vi "Edit Saquencer Array.vi"(11 "Sys Ini Path":path=path "D:/LABVIEW/SEQUENSER_SNA/Ver_12/INI/SysConfig.ini") -> ()   [LabVIEW 2018]
uses:
  Ctl/Step Type.ctl
  Ctl/MultiColumn Sequencer Table.ctl
  <vilib>/Utility/miscctls.llb/LVRowAndColumnUnsignedTypeDef.ctl
  <vilib>/Utility/miscctls.llb/LVRowAndColumnTypeDef.ctl
  Ctl/Test Step.ctl
  Ctl/Test Result.ctl
  Ctl/Sequencer Array.vi
  Ctl Main/Global Variable.vi
  <vilib>/Utility/config.llb/Read Key (String).vi
  <vilib>/Utility/config.llb/Read Key (U32).vi
  <vilib>/Utility/config.llb/Read Key (Double).vi
  <vilib>/Utility/config.llb/Read Key (Boolean).vi
  <vilib>/Utility/config.llb/Write Key (U32).vi
  <vilib>/Utility/config.llb/Write Key (String).vi
  <vilib>/Utility/config.llb/Write Key (Double).vi
  <vilib>/Utility/config.llb/Write Key (Boolean).vi
  <vilib>/Utility/config.llb/Write Key (I32).vi
  <vilib>/Utility/config.llb/NI_LVConfig.lvlib
panel:
  out "Sequencer File":string
  in  "Config":string="***"
  in  "Board":string="***"
  in  "Customer":string="***"
  in  "Sequencer\nExtend":bool
  in  "Save To File":bool
  in  "Load from File":bool
  in  "Value Nominal":dbl step=0.1 format="%#.3g"
  out "Row Selected":i16
  in  "Limits Calculate":bool
  in  "Test Sequencer":T1
  in  "New Step":bool
  in  "Measure Units":string
  in  "Remove Step":bool
  in  "Replace Step":bool
  in  "Insert Step":bool
  in  "Clear Array":bool
  in  "Exit Button":bool
  out "Steps":u16 max=500
  in  "Report":bool
  in  "Run/Skip":bool=TRUE
  in  "Parameters":string
  in  "Prc % (-)":i16=-5 min=-100 max=0 step=1
  in  "Prc % (+)":i16=5 min=0 max=100 step=1
  in  "Lower Limt":dbl step=0.1 format="%#.3g"
  in  "Upper Limt":dbl step=0.1 format="%#.3g"
  in  "Description":string
  in  "Step-ID":u16 max=255
  in  "Step Type":T2 items=["Label", "Settings", "Numeric", "String", "Boolean"]
  # "Step Editor"
  # "Nominal \nValue"
  # "Step Info"
  # "Measure Limits"
  # "File Operations"
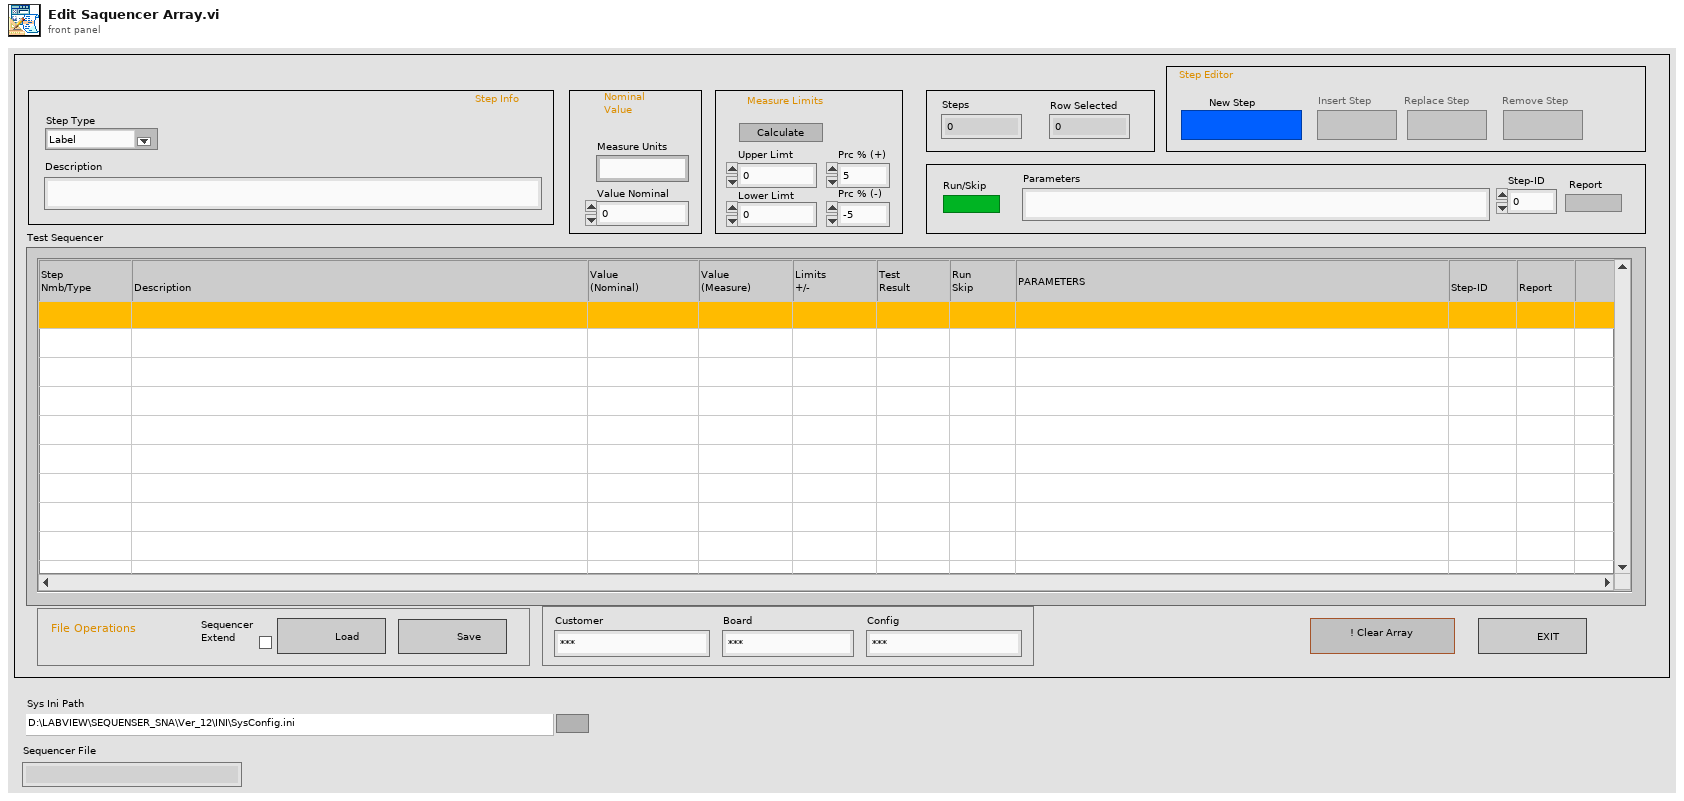
[diagram p1: front panel]
types:
  T1 = typedef "MultiColumn Sequencer Table.ctl" = i32
  T2 = typedef "Step Type.ctl" = u16
  T3 = typedef "LVRowAndColumnTypeDef.ctl" = cluster{"Row":i32, "Column":i32}
  T4 = typedef "LVRowAndColumnUnsignedTypeDef.ctl" = cluster{"Row":u32, "Column":u32}
  T5 = typedef "Test Step.ctl" = cluster{"Step ID":u16, "Step Description":string, "Step Type":u16, "Test Values":cluster{"Numeric Value":dbl, "Str Value":string, "Boolean Value":bool, "Upper Limit":dbl, "Lower Limit":dbl}, "Parameters":string, "Run/Skip":bool, "Test Result":T6, "Report":bool, "Measure Units":string}
  T6 = typedef "Test Result.ctl" = enum16{"Idle", "PASS", "FALSE"}
  T7 = enum8{"Enabled", "Disabled", "Disabled and Grayed Out"}
  T8 = enum16{"open", "replace", "create", "open or create", "replace or create", "replace or create with confirmation"}
  T9 = typedef "NI_LVConfig.lvlib/Config Data RefNum.ctl" = refnum<k1>
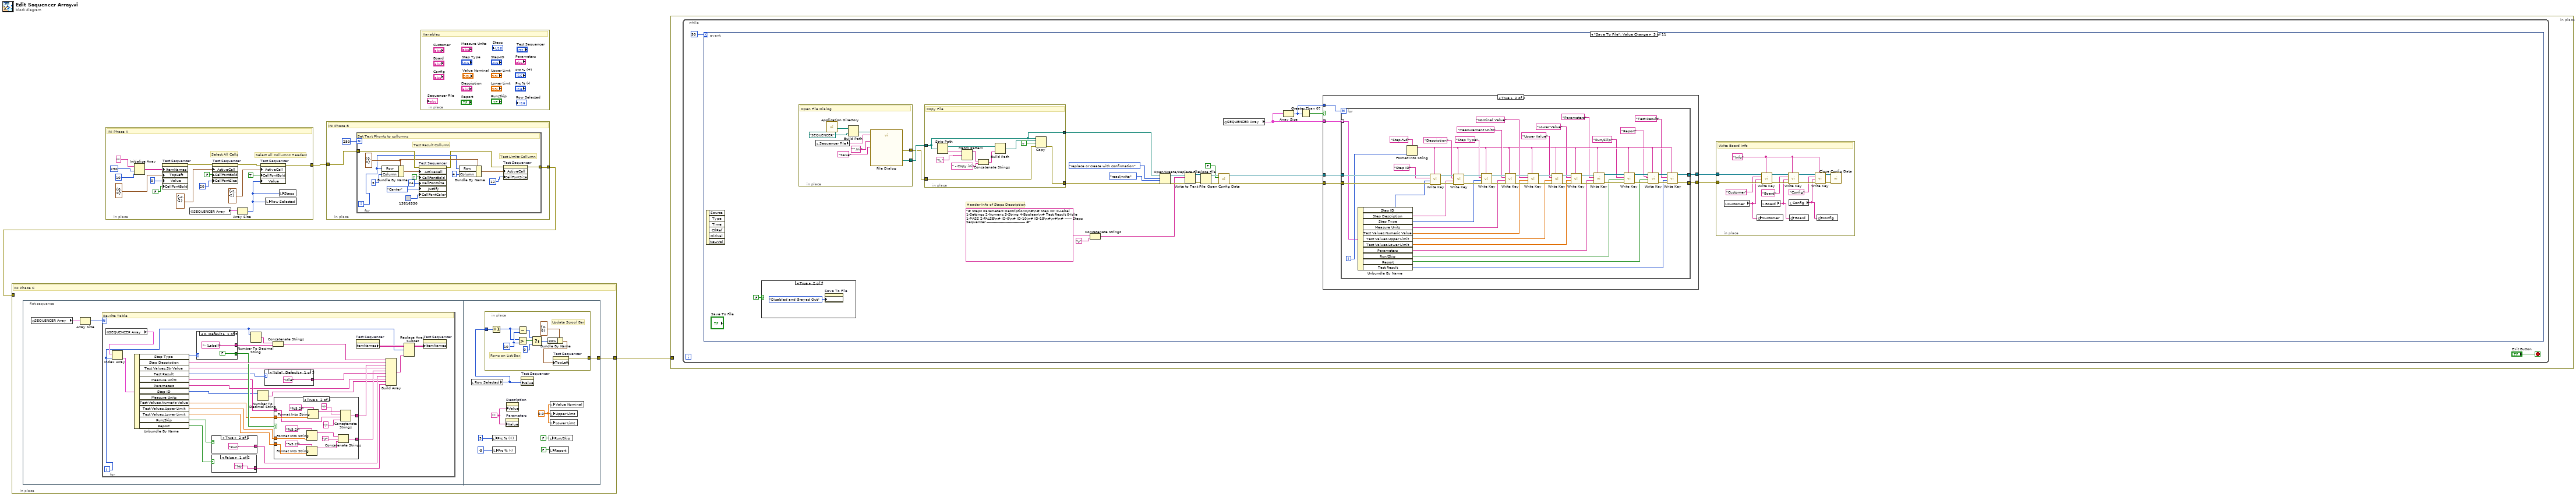
[diagram p0: block diagram]
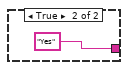
[diagram p2: hidden frame]
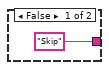
[diagram p3: hidden frame]
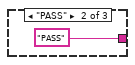
[diagram p4: hidden frame]
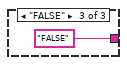
[diagram p5: hidden frame]
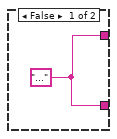
[diagram p6: hidden frame]
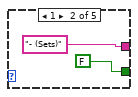
[diagram p7: hidden frame]
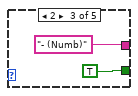
[diagram p8: hidden frame]
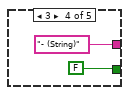
[diagram p9: hidden frame]
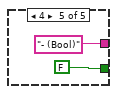
[diagram p10: hidden frame]
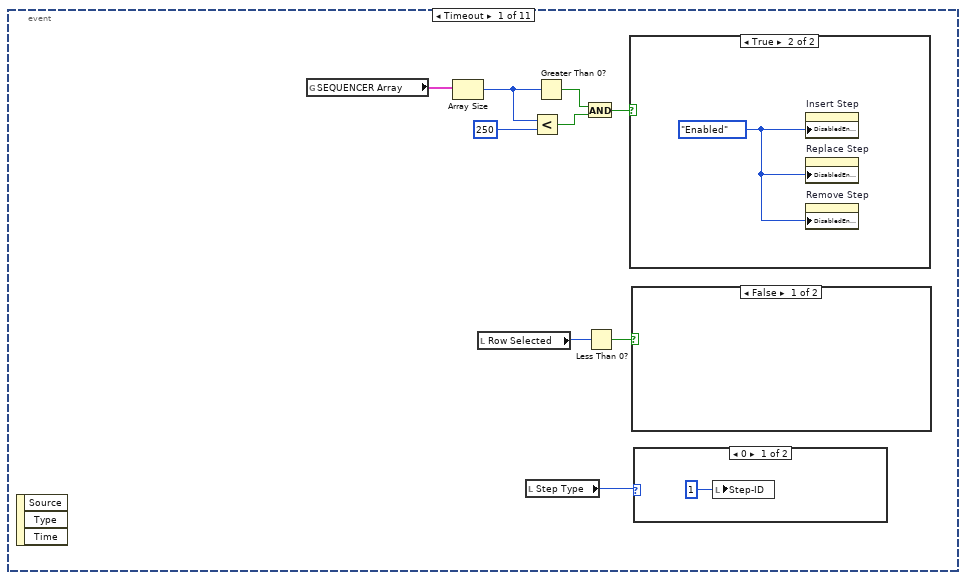
[diagram p11: hidden frame]
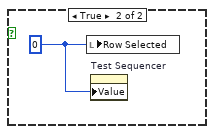
[diagram p13: hidden frame]
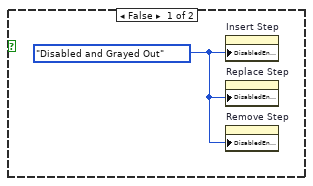
[diagram p14: hidden frame]
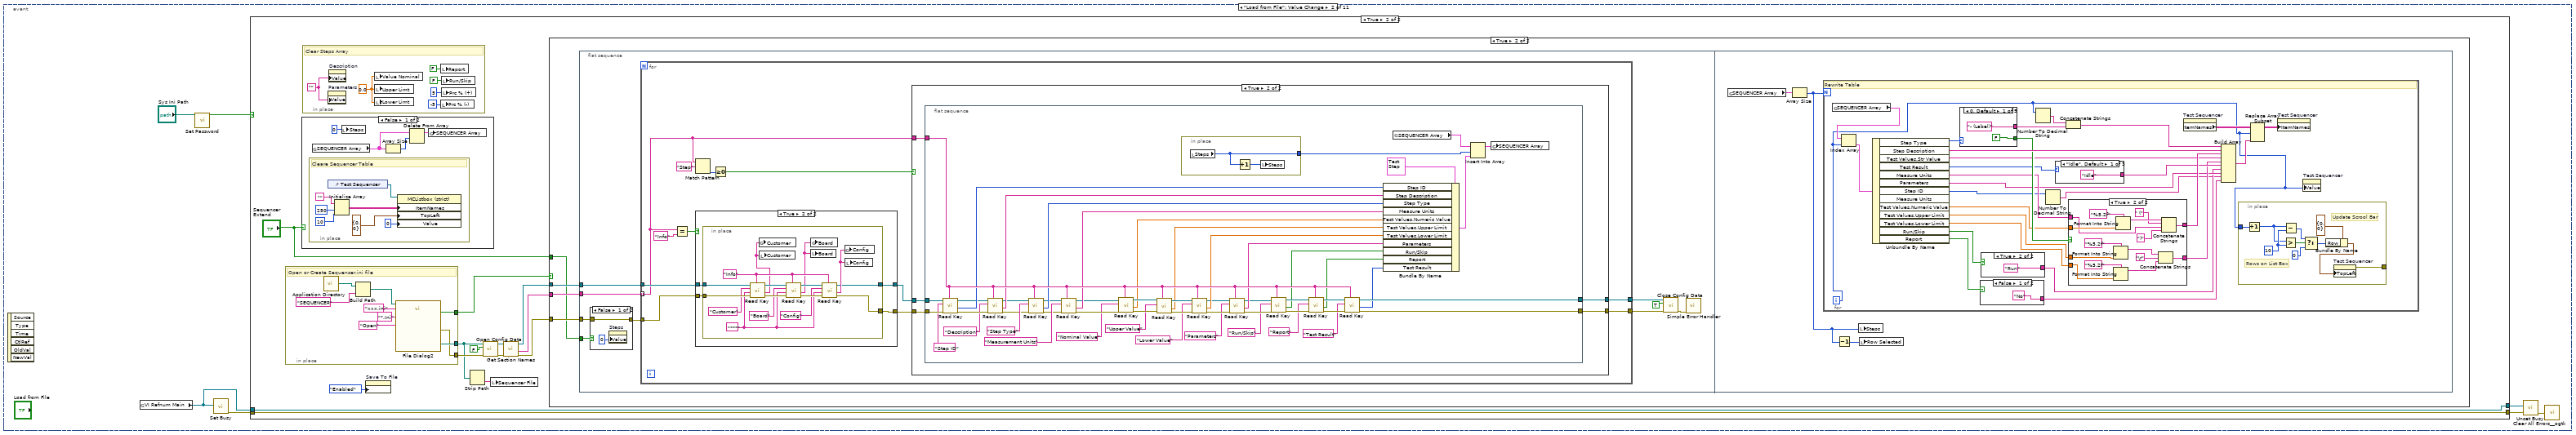
[diagram p15: hidden frame]
diagram:
  n1 = in-place {
    in-place-border: [w6] -> w3
    # "Select All Collumns Headers"
    # "Select All Cells"
    # "INI Phase A"
    n2 = Initialize Array("", 250 ("dimension size"), 10 ("dimension size")) -> (w18:string[][])
    n3 = property on="Test Sequencer" class="MCListbox (strict)"("ItemNames"=w18, "TopLeft"=T4 {"Row"=0, "Column"=0} ("Top Left Visible Cell"), "Value"=T1 0 ("Test Sequencer"), "CellFontBold"=FALSE ("Active Cell:Cell Font:Bold")) -> (error out=w13:errorcluster)  [unwired: 2 in, 1 out]
    n4 = global read "Sequencer Array.vi" "SEQUENCER Array"() -> (w5:T5[])
    n5 = property on="Test Sequencer" class="MCListbox (strict)"(error in=w13, "ActiveCell"=T3 {"Row"=-2, "Column"=-2} ("Active Cell:Active Cell"), "CellFontBold"=FALSE ("Active Cell:Cell Font:Bold"), "CellFontSize"=20 ("dimension size")) -> (error out=w7:errorcluster)  [unwired: 1 in, 1 out]
    n6 = Array Size(array=w5) -> (size(s)=w4:i32)
    n7 = property on="Test Sequencer" class="MCListbox (strict)"(error in=w7, "ActiveCell"=T3 {"Row"=-1, "Column"=-2} ("Active Cell:Active Cell"), "CellFontBold"=TRUE ("Active Cell:Cell Font:Bold"), "Value"=w4) -> (error out=w6:errorcluster)  [unwired: 1 in, 1 out]
    n8 = local write "Row Selected"(w4) -> ()
    n9 = local write "Steps"(w4) -> ()
  }
  n10 = in-place {
    in-place-border: w3 -> [w22]
    in-place-border: [w21] -> w2
    # "INI Phase B"
    n11 = for {
      N: 250 -> [_]
      tunnel: w22 -> [w35]
      tunnel: [w27] -> w21
      i -> [w28]
      w30 = T3 {"Row"=0, "Column"=0} ("Active Cell:Active Cell")
      # "Test Limits Collumn"
      # "Test Result Collumn"
      # "Set Text Phonts to collumns"
      n12 = Bundle By Name(cluster=w30, "Row"=w28, "Column"=5) -> (w37:T3)
      n13 = property on="Test Sequencer" class="MCListbox (strict)"(error in=w35, "ActiveCell"=w37, "CellFontBold"=TRUE ("Active Cell:Cell Font:Bold"), "CellFontSize"=u32 24 ("Active Cell:Cell Font:Size"), "Justify"=enum16{"Left", "Center", "Right"}."Center" ("Active Cell:Cell Justification"), "CellFontColor"=u32 13816530) -> (error out=w26:errorcluster)  [unwired: 1 in, 1 out]
      n14 = Bundle By Name(cluster=w30, "Row"=w28, "Column"=4) -> (w29:T3)
      n15 = property on="Test Sequencer" class="MCListbox (strict)"(error in=w26, "ActiveCell"=w29, "CellFontSize"=12 ("Column")) -> (error out=w27:errorcluster)  [unwired: 1 in, 1 out]
    }
  }
  n16 = in-place {
    in-place-border: w2 -> [_]
    in-place-border: [w38] -> w1
    # "INI Phase C"
    n17 = flat-sequence {
      tunnel: [w108] -> w38
      frame #0 {
        n18 = global read "Sequencer Array.vi" "SEQUENCER Array"() -> (w40:T5[])
        n19 = Array Size(array=w40) -> (size(s)=w39:i32)
        n20 = for {
          N: w39 -> [_]
          i -> [w63]
          # "Revrite Table"
          n21 = global read "Sequencer Array.vi" "SEQUENCER Array"() -> (w68:T5[])
          n22 = Index Array(array=w68, index=w63) -> (element=w49:T5)
          n23 = Unbundle By Name(w49) -> ("Step Type"=w67:u16, "Step Description"=w59:string, "Test Values.Str Value"=w55:string, "Test Result"=w54:T6, "Measure Units"=w52:string, "Parameters"=w48:string, "Step ID"=w50:u16, "Test Values.Numeric Value"=w57:dbl, "Test Values.Upper Limit"=w47:dbl, "Test Values.Lower Limit"=w46:dbl, "Run/Skip"=w45:bool, "Report"=w44:bool)  [unwired: 1 out]
          n24 = case shown="0, Default" w67 {
            tunnel: ["- (Label)" "- (Sets)" "- (Numb)" "- (String)" "- (Bool)"] -> w61
            tunnel: [FALSE FALSE TRUE FALSE FALSE] -> w58
            frame 0, Default {
            }
            frame 1 {
            }
            frame 2 {
            }
            frame 3 {
            }
            frame 4 {
            }
          }
          n25 = case shown="False" w44 {
            tunnel: ["No" "Yes"] -> w42
            frame False {
            }
            frame True {
            }
          }
          n26 = case shown="True" w45 {
            tunnel: ["Skip" "Run"] -> w43
            frame False {
            }
            frame True {
            }
          }
          n27 = Number To Decimal String(number=w63) -> (decimal integer string=w62:string)  [unwired: 1 in]
          n28 = Number To Decimal String(number=w50) -> (decimal integer string=w41:string)  [unwired: 1 in]
          n29 = case shown="\"Idle\", Default" w54 {
            tunnel: ["Idle" "PASS" "FALSE"] -> w53
            frame "Idle", Default {
            }
            frame "PASS" {
            }
            frame "FALSE" {
            }
          }
          n30 = Concatenate Strings(w62, w61) -> (w60:string)
          n31 = case shown="True" w58 {
            tunnel: [w76 w85] -> w51
            tunnel: [w76 w82] -> w56
            tunnel: w57 -> [_ w80]
            tunnel: w47 -> [_ w79]
            tunnel: w46 -> [_ w78]
            tunnel: w52 -> [_ w77]
            frame False {
              w76 = "..."
            }
            frame True {
              n32 = Format Into String(format string="%5.2f", w79) -> (resulting string=w87:string)  [unwired: 2 in, 1 out]
              n33 = Format Into String(format string="%5.2f", w78) -> (resulting string=w86:string)  [unwired: 2 in, 1 out]
              n34 = Format Into String(format string="%5.2f", w80) -> (resulting string=w84:string)  [unwired: 2 in, 1 out]
              n35 = Concatenate Strings(w87, "\r", w86) -> (w85:string)
              n36 = Concatenate Strings(w84, "(", w77, ")") -> (w82:string)
            }
          }
          n37 = property on="Test Sequencer" class="MCListbox (strict)"() -> ("ItemNames"=w66:string[][])  [unwired: 2 in, 2 out]
          n38 = Build Array(w60, w59, w56, w55, w51, w53, w43, w48, w41, w42) -> (w64:string[])
          n39 = Replace Array Subset(array=w66, new element=w64, index (row)=w63) -> (w65:string[][])  [unwired: 1 in]
          n40 = property on="Test Sequencer" class="MCListbox (strict)"("ItemNames"=w65) -> ()  [unwired: 2 in, 2 out]
        }
      }
      frame #1 {
        w106 = 0.0
        w107 = ""
        n41 = local read "Row Selected"() -> (w109:i16)
        n42 = in-place {
          in-place-border: w109 -> [w113]
          in-place-border: [w110] -> w108
          w115 = 10 ("y")
          # "Update Scrool Bar"
          # "Rows on List Box"
          n43 = Increment(x=w113) -> (x+1=w112:i16)
          n44 = Greater?(x=w112, y=w115) -> (0:w118:bool)
          n45 = Subtract(x=w112, y=w115) -> (x-y=w116:i32)
          n46 = Select(t=w116, s=w118, f=0) -> (s? t:f=w114:i32)
          n47 = Bundle By Name(cluster=T4 {"Row"=0, "Column"=0} ("Top Left Visible Cell"), "Row"=w114) -> (w111:T4)
          n48 = property on="Test Sequencer" class="MCListbox (strict)"("TopLeft"=w111) -> (error out=w110:errorcluster)  [unwired: 2 in, 1 out]
        }
        n49 = local write "Prc % (+)"(5) -> ()
        n50 = local write "Prc % (-)"(i16 -5 ("Prc % (-)")) -> ()
        n51 = property on="Parameters" class="Str"("Value"=w107) -> ()  [unwired: 2 in, 2 out]
        n52 = property on="Description" class="Str"("Value"=w107) -> ()  [unwired: 2 in, 2 out]
        n53 = property on="Test Sequencer" class="MCListbox (strict)"("Value"=w109) -> ()  [unwired: 2 in, 2 out]
        n54 = local write "Run/Skip"(FALSE ("Run/Skip")) -> ()
        n55 = local write "Report"(FALSE ("Report")) -> ()
        n56 = local write "Value Nominal"(w106) -> ()
        n57 = local write "Upper Limt"(w106) -> ()
        n58 = local write "Lower Limt"(w106) -> ()
      }
    }
  }
  n59 = in-place {
    # "Variables"
  }
  n60 = in-place {
    in-place-border: w1 -> [_]
    n61 = while {
      stop <- "Exit Button" stop-if-true
      n62 = event shown="[2] \"Save To File\": Value Change" {
        selector: _ -> [_ _ _ _ _ _ _ _ _ _ _]
        dyn-events: _ -> [_ _ _ _ _ _ _ _ _ _ _]
        timeout: 50 -> [_ _ _ _ _ _ _ _ _ _ _]
        event Timeout {
          n63 = event-data() -> ()  [unwired: 1 in, 3 out]
          n64 = global read "Sequencer Array.vi" "SEQUENCER Array"() -> (w130:T5[])
          n65 = Array Size(array=w130) -> (size(s)=w129:i32)
          n66 = local read "Row Selected"() -> (w124:i16)
          n67 = local read "Step Type"() -> (w122:T2)
          n68 = Less?(x=w129, y=250) -> (x < y?=w126:bool)
          n69 = Greater Than 0?(x=w129) -> (x > 0?=w127:bool)
          n70 = And(x=w127, y=w126) -> (x .and. y?=w125:bool)
          n71 = Less Than 0?(x=w124) -> (x < 0?=w123:bool)
          n72 = case shown="True" w125 {
            frame False {
              w133 = T7."Disabled and Grayed Out" ("Disabled")
              n73 = property on="Insert Step" class="Bool"("DisabledEnum"=w133) -> ()  [unwired: 2 in, 2 out]
              n74 = property on="Replace Step" class="Bool"("DisabledEnum"=w133) -> ()  [unwired: 2 in, 2 out]
              n75 = property on="Remove Step" class="Bool"("DisabledEnum"=w133) -> ()  [unwired: 2 in, 2 out]
            }
            frame True {
              w134 = T7."Enabled" ("Disabled")
              n76 = property on="Insert Step" class="Bool"("DisabledEnum"=w134) -> ()  [unwired: 2 in, 2 out]
              n77 = property on="Replace Step" class="Bool"("DisabledEnum"=w134) -> ()  [unwired: 2 in, 2 out]
              n78 = property on="Remove Step" class="Bool"("DisabledEnum"=w134) -> ()  [unwired: 2 in, 2 out]
            }
          }
          n79 = case shown="False" w123 {
            frame False {
            }
            frame True {
              w132 = u16 0 ("Row Selected")
              n80 = local write "Row Selected"(w132) -> ()
              n81 = property on="Test Sequencer" class="MCListbox (strict)"("Value"=w132) -> ()  [unwired: 2 in, 2 out]
            }
          }
          n82 = case shown="0" w122 {
            frame 0 {
              n83 = local write "Step-ID"(1) -> ()
            }
            frame 1, Default {
            }
          }
        }
        event "Load from File": Value Change {
          n84 = event-data() -> ()  [unwired: 1 in, 6 out]
          n85 = global read "Global Variable.vi" "VI Refnum Main"() -> (w135:refnum<vi>)
          n86 = call "Set Password.vi"("Ini File"="Sys Ini Path") -> ("Password Ok"=w140:bool)  [unwired: 9 in, 1 out]
          n87 = call <vilib>:"Set Busy.vi"("VI reference (current VI)"=w135) -> ("error out"=w139:errorcluster)  [unwired: 9 in, 1 out]
          n88 = case shown="True" w140 {
            tunnel: w139 -> [w143 w145]
            tunnel: [w143 w145] -> w138
            tunnel: w135 -> [w142 w144]
            tunnel: [w142 w144] -> w136
            frame False {
            }
            frame True {
              n89 = in-place {
                in-place-border: [w366] -> w150
                in-place-border: [w365] -> w147
                in-place-border: [w364] -> w157
                # "Open or Create Sequenser.ini file"
                n90 = call <vilib>:"Application Directory.vi"() -> ("Application Directory"=w361:path)
                n91 = Build Path(base path=w361, name or relative path="SEQUENCER") -> (appended path=w363:path)
                n92 = call "File Dialog2"("start path"=w363, "button label"="Open", "default name"="xxx.ini", "pattern (all files)"="*.Ini") -> ("selected path"=w365:path, "exists"=w366:bool, "error out"=w364:errorcluster)  [unwired: 8 in, 1 out]
              }
              n93 = case shown="False" "Sequencer\nExtend" {
                frame False {
                  n94 = in-place "In Place Element Structure" {
                    # "Cleare Sequencer Table"
                    n95 = control-ref of="Test Sequencer"() -> (w163:refnum<vi>)
                    n96 = Initialize Array("", 250 ("dimension size"), 10 ("dimension size")) -> (w166:string[][])
                    n97 = property on="Property Node" class="MCListbox (strict)"(reference=w163, "ItemNames"=w166, "TopLeft"=T4 {"Row"=0, "Column"=0} ("Top Left Visible Cell"), "Value"=T1 0 ("Test Sequencer")) -> ()  [unwired: 1 in, 2 out]
                  }
                  n98 = global read "Sequencer Array.vi" "SEQUENCER Array"() -> (w159:T5[])
                  n99 = local write "Steps"(u16 0 ("Steps")) -> ()
                  n100 = Array Size(array=w159) -> (size(s)=w160:i32)
                  n101 = Delete From Array(array=w159, length=w160) -> (array with subset deleted=w161:T5[])  [unwired: 1 in, 1 out]
                  n102 = global write "Sequencer Array.vi" "SEQUENCER Array"(w161) -> ()
                }
                frame True {
                }
              }
              n103 = in-place {
                w355 = 0.0
                w354 = ""
                # "Clear Steps Array"
                n104 = property on="Parameters" class="Str"("Value"=w354) -> ()  [unwired: 2 in, 2 out]
                n105 = property on="Description" class="Str"("Value"=w354) -> ()  [unwired: 2 in, 2 out]
                n106 = local write "Value Nominal"(w355) -> ()
                n107 = local write "Upper Limt"(w355) -> ()
                n108 = local write "Lower Limt"(w355) -> ()
                n109 = local write "Report"(FALSE ("Report")) -> ()
                n110 = local write "Prc % (-)"(i16 -5 ("Prc % (-)")) -> ()
                n111 = local write "Run/Skip"(FALSE ("Run/Skip")) -> ()
                n112 = local write "Prc % (+)"(5) -> ()
              }
              n113 = property on="Save To File" class="Bool"("DisabledEnum"=T7."Enabled" ("Disabled")) -> ()  [unwired: 2 in, 2 out]
              n114 = Strip Path(path=w147) -> (name=w146:string)  [unwired: 1 out]
              n115 = call <vilib>:"Open Config Data.vi"("error in (no error)"=w157, "create file if necessary (T)"=FALSE, "configuration file path"=w147) -> ("error out"=w154:errorcluster, "refnum"=w155:T9)  [unwired: 6 in, 1 out]
              n116 = local write "Sequencer File"(w146) -> ()
              n117 = call <vilib>:"Get Section Names.vi"("error in (no error)"=w154, "refnum"=w155) -> ("error out"=w151:errorcluster, "section names"=w152:string[], "refnum out"=w153:T9)  [unwired: 7 in]
              n118 = case shown="True" w150 {
                tunnel: w153 -> [_ w172]
                tunnel: w152 -> [_ w171]
                tunnel: w151 -> [_ w170]
                tunnel: "Sequencer\nExtend" -> [_ w169]
                frame False {
                }
                frame True {
                  n119 = flat-sequence {
                    tunnel: w172 -> [w176]
                    tunnel: w171 -> [w181]
                    tunnel: w170 -> [w174]
                    tunnel: w169 -> [w173]
                    frame #0 {
                      n120 = case shown="False" w173 {
                        tunnel: [w183 w184] -> w175
                        tunnel: w174 -> [w183 w184]
                        frame False {
                          n121 = property on="Steps" class="DigNum (strict)"("Value"=u16 0 ("Steps")) -> ()  [unwired: 2 in, 2 out]
                        }
                        frame True {
                        }
                      }
                      n122 = for {
                        tunnel: w181 -> [w188] mode=indexing
                        tunnel: w175 -> [w193]
                        tunnel: [w196] -> w178
                        tunnel: [w195] -> w177
                        tunnel: w176 -> [w194]
                        n123 = Equal?(x=w188, y="Info") -> (x = y?=w189:bool)
                        n124 = Match Pattern(string=w188, regular expression="Step") -> (offset past match=w186:i32)  [unwired: 1 in, 3 out]
                        n125 = case shown="True" w189 {
                          tunnel: w194 -> [w259 w263]
                          tunnel: w193 -> [w258 w262]
                          tunnel: [w259 w261] -> w192
                          tunnel: [w258 w260] -> w191
                          frame False {
                          }
                          frame True {
                            n126 = in-place {
                              in-place-border: w263 -> [w275]
                              in-place-border: w262 -> [w274]
                              in-place-border: [w265] -> w261
                              in-place-border: [w264] -> w260
                              w269 = "***"
                              w273 = "Info"
                              n127 = call-poly <vilib>:"Read Key.vi"("section"=w273, "error in (no error)"=w274, "default value"=w269, "key"="Customer", "refnum"=w275) -> ("error out"=w278:errorcluster, "value"=w266:string, "refnum out"=w276:T9)  [unwired: 3 in, 1 out]
                              n128 = global write "Global Variable.vi" "Customer"(w266) -> ()
                              n129 = local write "Customer"(w266) -> ()
                              n130 = call-poly <vilib>:"Read Key.vi"("section"=w273, "error in (no error)"=w278, "default value"=w269, "key"="Board", "refnum"=w276) -> ("error out"=w279:errorcluster, "value"=w268:string, "refnum out"=w277:T9)  [unwired: 3 in, 1 out]
                              n131 = global write "Global Variable.vi" "Board"(w268) -> ()
                              n132 = local write "Board"(w268) -> ()
                              n133 = call-poly <vilib>:"Read Key.vi"("section"=w273, "error in (no error)"=w279, "default value"=w269, "key"="Config", "refnum"=w277) -> ("error out"=w264:errorcluster, "value"=w267:string, "refnum out"=w265:T9)  [unwired: 3 in, 1 out]
                              n134 = global write "Global Variable.vi" "Config"(w267) -> ()
                              n135 = local write "Config"(w267) -> ()
                            }
                          }
                        }
                        n136 = Greater Or Equal To 0?(x=w186) -> (x >= 0?=w185:bool)
                        n137 = case shown="True" w185 {
                          tunnel: [w198 w203] -> w196
                          tunnel: [w197 w202] -> w195
                          tunnel: w192 -> [w198 w201]
                          tunnel: w191 -> [w197 w200]
                          tunnel: w188 -> [_ w199]
                          frame False {
                          }
                          frame True {
                            n138 = flat-sequence {
                              tunnel: [w254] -> w202
                              tunnel: [w255] -> w203
                              tunnel: w199 -> [w251]
                              tunnel: w200 -> [w252]
                              tunnel: w201 -> [w253]
                              frame #0 {
                                n139 = call-poly <vilib>:"Read Key.vi"("section"=w251, "error in (no error)"=w252, "key"="Step ID", "refnum"=w253) -> ("error out"=w243:errorcluster, "value"=w245:u32, "refnum out"=w244:T9)  [unwired: 4 in, 1 out]
                                n140 = call-poly <vilib>:"Read Key.vi"("section"=w251, "error in (no error)"=w243, "key"="Description", "refnum"=w244) -> ("error out"=w238:errorcluster, "value"=w241:string, "refnum out"=w239:T9)  [unwired: 4 in, 1 out]
                                n141 = call-poly <vilib>:"Read Key.vi"("section"=w251, "error in (no error)"=w238, "key"="Step Type", "refnum"=w239) -> ("error out"=w234:errorcluster, "value"=w237:u32, "refnum out"=w235:T9)  [unwired: 4 in, 1 out]
                                n142 = call-poly <vilib>:"Read Key.vi"("section"=w251, "error in (no error)"=w234, "key"="Measurement Units", "refnum"=w235) -> ("error out"=w229:errorcluster, "value"=w233:string, "refnum out"=w232:T9)  [unwired: 4 in, 1 out]
                                n143 = call-poly <vilib>:"Read Key.vi"("section"=w251, "error in (no error)"=w229, "key"="Nominal Value", "refnum"=w232) -> ("error out"=w228:errorcluster, "value"=w223:dbl, "refnum out"=w231:T9)  [unwired: 4 in, 1 out]
                                n144 = call-poly <vilib>:"Read Key.vi"("section"=w251, "error in (no error)"=w228, "key"="Upper Value", "refnum"=w231) -> ("error out"=w227:errorcluster, "value"=w222:dbl, "refnum out"=w230:T9)  [unwired: 4 in, 1 out]
                                n145 = in-place {
                                in-place-border: [w257] -> w204
                                n146 = local read "Steps"() -> (w257:u16)
                                n147 = Increment(x=w257) -> (x+1=w256:u16)
                                n148 = local write "Steps"(w256) -> ()
                                }
                                n149 = call-poly <vilib>:"Read Key.vi"("section"=w251, "error in (no error)"=w227, "key"="Lower Value", "refnum"=w230) -> ("error out"=w219:errorcluster, "value"=w221:dbl, "refnum out"=w220:T9)  [unwired: 4 in, 1 out]
                                n150 = call-poly <vilib>:"Read Key.vi"("section"=w251, "error in (no error)"=w219, "key"="Parameters", "refnum"=w220) -> ("error out"=w213:errorcluster, "value"=w217:string, "refnum out"=w216:T9)  [unwired: 4 in, 1 out]
                                n151 = call-poly <vilib>:"Read Key.vi"("section"=w251, "error in (no error)"=w213, "key"="Run/Skip", "refnum"=w216) -> ("error out"=w212:errorcluster, "value"=w209:bool, "refnum out"=w215:T9)  [unwired: 4 in, 1 out]
                                n152 = call-poly <vilib>:"Read Key.vi"("section"=w251, "error in (no error)"=w212, "key"="Report", "refnum"=w215) -> ("error out"=w211:errorcluster, "value"=w206:bool, "refnum out"=w214:T9)  [unwired: 4 in, 1 out]
                                n153 = call-poly <vilib>:"Read Key.vi"("section"=w251, "error in (no error)"=w211, "key"="Test Result", "refnum"=w214) -> ("error out"=w254:errorcluster, "value"=w205:u32, "refnum out"=w255:T9)  [unwired: 4 in, 1 out]
                                n154 = Bundle By Name(cluster=T5 {"Step ID"=0, "Step Description"="", "Step Type"=0, "Test Values"={"Numeric Value"=0.0, "Str Value"="", "Boolean Value"=TRUE, "Upper Limit"=0.0, "Lower Limit"=0.0}, "Parameters"="", "Run/Skip"=TRUE, "Test Result"=enum."Idle", "Report"=TRUE, "Measure Units"="..."} ("Test Step"), "Step ID"=w245, "Step Description"=w241, "Step Type"=w237, "Measure Units"=w233, "Test Values.Numeric Value"=w223, "Test Values.Upper Limit"=w222, "Test Values.Lower Limit"=w221, "Parameters"=w217, "Run/Skip"=w209, "Report"=w206, "Test Result"=w205) -> (w247:T5)
                                n155 = global read "Sequencer Array.vi" "SEQUENCER Array"() -> (w250:T5[])
                                n156 = Insert Into Array(array=w250, index=w204, new element=w247) -> (w249:T5[])
                                n157 = global write "Sequencer Array.vi" "SEQUENCER Array"(w249) -> ()
                              }
                            }
                          }
                        }
                      }
                      n158 = call <vilib>:"Close Config Data.vi"("error in (no error)"=w177, "write file if changed (T)"=TRUE, "refnum"=w178) -> ("error out"=w179:errorcluster)  [unwired: 7 in, 1 out]
                      n159 = call <vilib>:"Simple Error Handler.vi"("error in (no error)"=w179) -> ()  [unwired: 4 in, 5 out]
                    }
                    frame #1 {
                      n160 = global read "Sequencer Array.vi" "SEQUENCER Array"() -> (w280:T5[])
                      n161 = Array Size(array=w280) -> (size(s)=w281:i32)
                      n162 = for {
                        N: w281 -> [_]
                        i -> [w283]
                        # "Rewrite Table"
                        n163 = global read "Sequencer Array.vi" "SEQUENCER Array"() -> (w310:T5[])
                        n164 = Index Array(array=w310, index=w283) -> (element=w292:T5)
                        n165 = Unbundle By Name(w292) -> ("Step Type"=w309:u16, "Step Description"=w302:string, "Test Values.Str Value"=w298:string, "Test Result"=w297:T6, "Measure Units"=w295:string, "Parameters"=w291:string, "Step ID"=w293:u16, "Test Values.Numeric Value"=w300:dbl, "Test Values.Upper Limit"=w290:dbl, "Test Values.Lower Limit"=w289:dbl, "Run/Skip"=w288:bool, "Report"=w287:bool)  [unwired: 1 out]
                        n166 = case shown="0, Default" w309 {
                          tunnel: ["- (Label)" "- (Sets)" "- (Numb)" "- (String)" "- (Bool)"] -> w304
                          tunnel: [FALSE FALSE TRUE FALSE FALSE] -> w301
                          frame 0, Default {
                          }
                          frame 1 {
                          }
                          frame 2 {
                          }
                          frame 3 {
                          }
                          frame 4 {
                          }
                        }
                        n167 = case shown="False" w287 {
                          tunnel: ["No" "Yes"] -> w285
                          frame False {
                          }
                          frame True {
                          }
                        }
                        n168 = case shown="True" w288 {
                          tunnel: ["Skip" "Run"] -> w286
                          frame False {
                          }
                          frame True {
                          }
                        }
                        n169 = Number To Decimal String(number=w283) -> (decimal integer string=w305:string)  [unwired: 1 in]
                        n170 = Number To Decimal String(number=w293) -> (decimal integer string=w284:string)  [unwired: 1 in]
                        n171 = case shown="\"Idle\", Default" w297 {
                          tunnel: ["Idle" "PASS" "FALSE"] -> w296
                          frame "Idle", Default {
                          }
                          frame "PASS" {
                          }
                          frame "FALSE" {
                          }
                        }
                        n172 = Concatenate Strings(w305, w304) -> (w303:string)
                        n173 = case shown="True" w301 {
                          tunnel: [w328 w337] -> w294
                          tunnel: [w328 w334] -> w299
                          tunnel: w300 -> [_ w332]
                          tunnel: w290 -> [_ w331]
                          tunnel: w289 -> [_ w330]
                          tunnel: w295 -> [_ w329]
                          frame False {
                            w328 = "..."
                          }
                          frame True {
                            n174 = Format Into String(format string="%5.2f", w331) -> (resulting string=w339:string)  [unwired: 2 in, 1 out]
                            n175 = Format Into String(format string="%5.2f", w330) -> (resulting string=w338:string)  [unwired: 2 in, 1 out]
                            n176 = Format Into String(format string="%5.2f", w332) -> (resulting string=w336:string)  [unwired: 2 in, 1 out]
                            n177 = Concatenate Strings(w339, "\r", w338) -> (w337:string)
                            n178 = Concatenate Strings(w336, " (", w329, ")") -> (w334:string)
                          }
                        }
                        n179 = property on="Test Sequencer" class="MCListbox (strict)"() -> ("ItemNames"=w308:string[][])  [unwired: 2 in, 2 out]
                        n180 = Build Array(w303, w302, w299, w298, w294, w296, w286, w291, w284, w285) -> (w306:string[])
                        n181 = in-place {
                          in-place-border: w283 -> [w314]
                          in-place-border: [w311] -> _
                          w316 = 10 ("y")
                          # "Update Scrool Bar"
                          # "Rows on List Box"
                          n182 = Increment(x=w314) -> (x+1=w313:i32)
                          n183 = Greater?(x=w313, y=w316) -> (0:w319:bool)
                          n184 = Subtract(x=w313, y=w316) -> (x-y=w317:i32)
                          n185 = Select(t=w317, s=w319, f=0) -> (s? t:f=w315:i32)
                          n186 = Bundle By Name(cluster=T4 {"Row"=0, "Column"=0} ("Top Left Visible Cell"), "Row"=w315) -> (w312:T4)
                          n187 = property on="Test Sequencer" class="MCListbox (strict)"("TopLeft"=w312) -> (error out=w311:errorcluster)  [unwired: 2 in, 1 out]
                        }
                        n188 = Replace Array Subset(array=w308, new element=w306, index (row)=w283) -> (w307:string[][])  [unwired: 1 in]
                        n189 = property on="Test Sequencer" class="MCListbox (strict)"("ItemNames"=w307) -> ()  [unwired: 2 in, 2 out]
                        n190 = property on="Test Sequencer" class="MCListbox (strict)"("Value"=w283) -> ()  [unwired: 2 in, 2 out]
                      }
                      n191 = Decrement(x=w281) -> (x-1=w282:i32)
                      n192 = local write "Steps"(w281) -> ()
                      n193 = local write "Row Selected"(w282) -> ()
                    }
                  }
                }
              }
            }
          }
          n194 = call <vilib>:"Unset Busy.vi"("error in (no error)"=w138, "VI reference (current VI)"=w136) -> ("error out"=w137:errorcluster)  [unwired: 9 in]
          n195 = call <userlib>:"Clear All Errors__ogtk.vi"("Error In"=w137) -> ()  [unwired: 3 in, 1 out]
        }
        event "Save To File": Value Change {
          # "Header Info of Steps Description"
          n196 = event-data() -> ()  [unwired: 1 in, 6 out]
          n197 = case shown="True" FALSE {
            frame False {
            }
            frame True {
              n198 = property on="Save To File" class="Bool"("DisabledEnum"=T7."Disabled and Grayed Out" ("Disabled")) -> ()  [unwired: 2 in, 2 out]
            }
          }
          n199 = in-place {
            in-place-border: [w397] -> w371
            in-place-border: [w396] -> w370
            # "Open File Dialog"
            n200 = local read "Sequencer File"() -> (w394:string)
            n201 = call <vilib>:"Application Directory.vi"() -> ("Application Directory"=w395:path)
            n202 = Build Path(base path=w395, name or relative path=path "SEQUENCER") -> (appended path=w399:path)
            n203 = call "File Dialog"("start path"=w399, "button label"="Save", "default name"=w394, "pattern (all files)"="*.Ini") -> ("selected path"=w397:path, "error out"=w396:errorcluster)  [unwired: 8 in, 2 out]
          }
          n204 = in-place {
            in-place-border: [w404] -> w372
            in-place-border: w371 -> [w404]
            in-place-border: w370 -> [w403]
            in-place-border: [w402] -> w369
            # "Copy File"
            n205 = Strip Path(path=w404) -> (stripped path=w408:path, name=w401:string)
            n206 = Match Pattern(string=w401, regular expression="\\.") -> (before substring=w410:string)  [unwired: 1 in, 3 out]
            n207 = Concatenate Strings(w410, " - Copy.ini" ("string")) -> (w409:string)
            n208 = Build Path(base path=w408, name or relative path=w409) -> (appended path=w407:path)
            n209 = Copy(8:w403, 9:TRUE ("overwrite (F)"), 10:w407, 11:w404) -> (0:w402:errorcluster)  [unwired: 1 in, 2 out]
          }
          n210 = Concatenate Strings("# Steps Parameters Descriptions\n#\n# Step ID: 0-Label 1-Settings 2-Numeric 3-String 4-Boolean\n# Test Result 0-Idle 1-PASS 2-FALSE\n# ID-0\n# ID-10\n# ID-15\n#\n#\n# ------ Steps Sequenser --------------------------------- #" ("text"), "\r") -> (w375:string)
          n211 = Open/Create/Replace File(file path (use dialog)=w372, error in=w369, operation (0:open)=T8."replace or create with confirmation", access (0:read/write)=enum16{"read/write", "read-only", "write-only"}."read/write") -> (refnum out=w392:refnum<file>, error out=w391:errorcluster)  [unwired: 2 in, 1 out]
          n212 = Write to Text File(file (use dialog)=w392, text=w375, error in=w391) -> (refnum out=w389:refnum<file>, error out=w388:errorcluster)  [unwired: 1 in, 1 out]
          n213 = Close File(refnum=w389, error in=w388) -> (path=w386:path, error out=w387:errorcluster)
          n214 = call <vilib>:"Open Config Data.vi"("error in (no error)"=w387, "create file if necessary (T)"=FALSE, "configuration file path"=w386) -> ("error out"=w384:errorcluster, "refnum"=w385:T9)  [unwired: 6 in, 1 out]
          n215 = global read "Sequencer Array.vi" "SEQUENCER Array"() -> (w379:T5[])
          n216 = Array Size(array=w379) -> (size(s)=w377:i32)
          n217 = Greater Than 0?(x=w377) -> (x > 0?=w378:bool)
          n218 = case shown="True" w378 {
            tunnel: w385 -> [w414 w420]
            tunnel: w384 -> [w413 w419]
            tunnel: [w414 w418] -> w381
            tunnel: [w413 w417] -> w380
            tunnel: w379 -> [_ w416]
            tunnel: w377 -> [_ w415]
            frame False {
            }
            frame True {
              n219 = for {
                N: w415 -> [_]
                tunnel: w419 -> [w469]
                tunnel: w420 -> [w470]
                tunnel: w416 -> [w463] mode=indexing
                tunnel: [w430] -> w418
                tunnel: [w435] -> w417
                i -> [w465]
                n220 = Unbundle By Name(w463) -> ("Step ID"=w462:u16, "Step Description"=w460:string, "Step Type"=w456:u16, "Measure Units"=w453:string, "Test Values.Numeric Value"=w445:dbl, "Test Values.Upper Limit"=w444:dbl, "Test Values.Lower Limit"=w443:dbl, "Parameters"=w428:string, "Run/Skip"=w427:bool, "Report"=w426:bool, "Test Result"=w425:T6)
                n221 = Format Into String(format string="Step-%d", w465) -> (resulting string=w429:string)  [unwired: 2 in, 1 out]
                n222 = call-poly <vilib>:"Write Key.vi"("section"=w429, "error in (no error)"=w469, "value"=w462, "key"="Step ID", "refnum"=w470) -> ("error out"=w467:errorcluster, "refnum out"=w468:T9)  [unwired: 4 in, 1 out]
                n223 = call-poly <vilib>:"Write Key.vi"("section"=w429, "error in (no error)"=w467, "value"=w460, "key"="Description", "refnum"=w468) -> ("error out"=w458:errorcluster, "refnum out"=w459:T9)  [unwired: 4 in, 1 out]
                n224 = call-poly <vilib>:"Write Key.vi"("section"=w429, "error in (no error)"=w458, "value"=w456, "key"="Step Type", "refnum"=w459) -> ("error out"=w454:errorcluster, "refnum out"=w455:T9)  [unwired: 4 in, 1 out]
                n225 = call-poly <vilib>:"Write Key.vi"("section"=w429, "error in (no error)"=w454, "value"=w453, "key"="Measurement Units", "refnum"=w455) -> ("error out"=w448:errorcluster, "refnum out"=w451:T9)  [unwired: 4 in, 1 out]
                n226 = call-poly <vilib>:"Write Key.vi"("section"=w429, "error in (no error)"=w448, "value"=w445, "key"="Nominal Value", "refnum"=w451) -> ("error out"=w447:errorcluster, "refnum out"=w450:T9)  [unwired: 4 in, 1 out]
                n227 = call-poly <vilib>:"Write Key.vi"("section"=w429, "error in (no error)"=w447, "value"=w444, "key"="Upper Value", "refnum"=w450) -> ("error out"=w446:errorcluster, "refnum out"=w449:T9)  [unwired: 4 in, 1 out]
                n228 = call-poly <vilib>:"Write Key.vi"("section"=w429, "error in (no error)"=w446, "value"=w443, "key"="Lower Value", "refnum"=w449) -> ("error out"=w439:errorcluster, "refnum out"=w434:T9)  [unwired: 4 in, 1 out]
                n229 = call-poly <vilib>:"Write Key.vi"("section"=w429, "error in (no error)"=w439, "value"=w428, "key"="Parameters", "refnum"=w434) -> ("error out"=w438:errorcluster, "refnum out"=w433:T9)  [unwired: 4 in, 1 out]
                n230 = call-poly <vilib>:"Write Key.vi"("section"=w429, "error in (no error)"=w438, "value"=w427, "key"="Run/Skip", "refnum"=w433) -> ("error out"=w437:errorcluster, "refnum out"=w432:T9)  [unwired: 4 in, 1 out]
                n231 = call-poly <vilib>:"Write Key.vi"("section"=w429, "error in (no error)"=w437, "value"=w426, "key"="Report", "refnum"=w432) -> ("error out"=w436:errorcluster, "refnum out"=w431:T9)  [unwired: 4 in, 1 out]
                n232 = call-poly <vilib>:"Write Key.vi"("section"=w429, "error in (no error)"=w436, "value"=w425, "key"="Test Result", "refnum"=w431) -> ("error out"=w435:errorcluster, "refnum out"=w430:T9)  [unwired: 4 in, 1 out]
              }
            }
          }
          n233 = in-place {
            in-place-border: w381 -> [w485]
            in-place-border: w380 -> [w484]
            w477 = "Info"
            # "Write Board Info"
            n234 = local read "Customer"() -> (w471:string)
            n235 = global write "Global Variable.vi" "Customer"(w471) -> ()
            n236 = call-poly <vilib>:"Write Key.vi"("section"=w477, "error in (no error)"=w484, "value"=w471, "key"="Customer", "refnum"=w485) -> ("error out"=w482:errorcluster, "refnum out"=w483:T9)  [unwired: 4 in, 1 out]
            n237 = local read "Board"() -> (w473:string)
            n238 = call-poly <vilib>:"Write Key.vi"("section"=w477, "error in (no error)"=w482, "value"=w473, "key"="Board", "refnum"=w483) -> ("error out"=w478:errorcluster, "refnum out"=w481:T9)  [unwired: 4 in, 1 out]
            n239 = local read "Config"() -> (w472:string)
            n240 = global write "Global Variable.vi" "Board"(w473) -> ()
            n241 = call-poly <vilib>:"Write Key.vi"("section"=w477, "error in (no error)"=w478, "value"=w472, "key"="Config", "refnum"=w481) -> ("error out"=w479:errorcluster, "refnum out"=w480:T9)  [unwired: 4 in, 1 out]
            n242 = global write "Global Variable.vi" "Config"(w472) -> ()
            n243 = call <vilib>:"Close Config Data.vi"("error in (no error)"=w479, "refnum"=w480) -> ()  [unwired: 8 in, 2 out]
          }
        }
        event Value Change {
          n244 = event-data() -> ("NewVal"=w486:T2)  [unwired: 1 in, 5 out]
          n245 = case shown="4" w486 {
            frame 0, Default {
              w487 = 0.0
              n246 = local write "Measure Units"("..." ("Measure Units")) -> ()
              n247 = local write "Value Nominal"(w487) -> ()
              n248 = local write "Upper Limt"(w487) -> ()
              n249 = local write "Lower Limt"(w487) -> ()
            }
            frame 1 {
              w489 = 0.0
              n250 = local write "Measure Units"("..." ("Measure Units")) -> ()
              n251 = local write "Upper Limt"(w489) -> ()
              n252 = local write "Lower Limt"(w489) -> ()
              n253 = local write "Value Nominal"(w489) -> ()
            }
            frame 2 {
              w491 = 0.0
              n254 = local write "Measure Units"("???" ("Measure Units")) -> ()
              n255 = local write "Upper Limt"(w491) -> ()
              n256 = local write "Lower Limt"(w491) -> ()
              n257 = local write "Value Nominal"(w491) -> ()
            }
            frame 3 {
              w493 = 0.0
              n258 = local write "Measure Units"("Str" ("Measure Units")) -> ()
              n259 = local write "Upper Limt"(w493) -> ()
              n260 = local write "Lower Limt"(w493) -> ()
              n261 = local write "Value Nominal"(w493) -> ()
            }
            frame 4 {
              w495 = 0.0
              n262 = local write "Measure Units"("Bool" ("Measure Units")) -> ()
              n263 = local write "Value Nominal"(w495) -> ()
              n264 = local write "Upper Limt"(w495) -> ()
              n265 = local write "Lower Limt"(w495) -> ()
            }
          }
        }
        event "Limits Calculate": Value Change {
          n266 = event-data() -> ()  [unwired: 1 in, 6 out]
          n267 = local read "Step Type"() -> (w497:T2)
          n268 = case shown="3" w497 {
            tunnel: [w500 w502 w505 w515 w517] -> w499
            tunnel: [w500 w502 w504 w515 w517] -> w498
            frame 0, Default {
              w500 = 0.0
            }
            frame 1 {
              w502 = 0.0
              n269 = local write "Value Nominal"(0.0) -> ()
            }
            frame 2 {
              # "Numeric Limmit Calculation"
              n270 = local read "Value Nominal"() -> (w503:dbl)
              n271 = local read "Prc % (+)"() -> (w511:i16)
              n272 = local read "Prc % (-)"() -> (w508:i16)
              n273 = Divide(x=w503, y=100.0) -> (x/y=w512:dbl)
              n274 = Divide(x=w503, y=100.0) -> (x/y=w510:dbl)
              n275 = Multiply(x=w512, y=w511) -> (x*y=w507:dbl)
              n276 = Multiply(x=w510, y=w508) -> (x*y=w506:dbl)
              n277 = Add(x=w503, y=w507) -> (x+y=w505:dbl)
              n278 = Add(x=w503, y=w506) -> (x+y=w504:dbl)
            }
            frame 3 {
              w515 = 0.0
              n279 = local write "Value Nominal"(0.0) -> ()
            }
            frame 4 {
              w517 = 0.0
              n280 = local write "Value Nominal"(0.0) -> ()
            }
          }
          n281 = local write "Upper Limt"(w499) -> ()
          n282 = local write "Lower Limt"(w498) -> ()
        }
        event "Insert Step": Value Change {
          n283 = event-data() -> ()  [unwired: 1 in, 6 out]
          n284 = flat-sequence {
            tunnel: [w519] -> w518
            tunnel: w518 -> [w539]
            frame #0 {
              n285 = local read "Step-ID"() -> (w525:u16)
              n286 = local read "Description"() -> (w526:string)
              n287 = local read "Step Type"() -> (w528:T2)
              n288 = local read "Parameters"() -> (w527:string)
              n289 = local read "Run/Skip"() -> (w529:bool)
              n290 = local read "Report"() -> (w530:bool)
              n291 = local read "Measure Units"() -> (w531:string)
              n292 = local read "Value Nominal"() -> (w537:dbl)
              n293 = local read "Upper Limt"() -> (w532:dbl)
              n294 = local read "Lower Limt"() -> (w533:dbl)
              n295 = Bundle By Name(cluster=T5 {"Step ID"=0, "Step Description"="", "Step Type"=0, "Test Values"={"Numeric Value"=0.0, "Str Value"="", "Boolean Value"=TRUE, "Upper Limit"=0.0, "Lower Limit"=0.0}, "Parameters"="", "Run/Skip"=TRUE, "Test Result"=enum."Idle", "Report"=TRUE, "Measure Units"="..."} ("Test Step"), "Step ID"=w525, "Step Description"=w526, "Step Type"=w528, "Parameters"=w527, "Run/Skip"=w529, "Report"=w530, "Measure Units"=w531, "Test Values.Numeric Value"=w537, "Test Values.Str Value"="<...>", "Test Values.Boolean Value"=TRUE, "Test Values.Upper Limit"=w532, "Test Values.Lower Limit"=w533, "Test Result"=Test_Result."Idle") -> (w523:T5)
              n296 = local read "Row Selected"() -> (w521:i16)
              n297 = global read "Sequencer Array.vi" "SEQUENCER Array"() -> (w524:T5[])
              n298 = Increment(x=w521) -> (x+1=w520:i16)
              n299 = Insert Into Array(array=w524, index=w520, new element=w523) -> (w522:T5[])
              n300 = Array Size(array=w522) -> (size(s)=w519:i32)
              n301 = global write "Sequencer Array.vi" "SEQUENCER Array"(w522) -> ()
              n302 = local write "Steps"(w519) -> ()
            }
            frame #1 {
              n303 = for {
                N: w539 -> [_]
                i -> [w562]
                # "Revrite Table"
                n304 = global read "Sequencer Array.vi" "SEQUENCER Array"() -> (w567:T5[])
                n305 = Index Array(array=w567, index=w562) -> (element=w548:T5)
                n306 = Unbundle By Name(w548) -> ("Step Type"=w566:u16, "Step Description"=w558:string, "Test Values.Str Value"=w554:string, "Test Result"=w553:T6, "Measure Units"=w551:string, "Parameters"=w547:string, "Step ID"=w549:u16, "Test Values.Numeric Value"=w556:dbl, "Test Values.Upper Limit"=w546:dbl, "Test Values.Lower Limit"=w545:dbl, "Run/Skip"=w544:bool, "Report"=w543:bool)  [unwired: 1 out]
                n307 = case shown="2" w566 {
                  tunnel: ["- (Label)" "- (Sets)" "- (Numer)" "- (String)" "- (Bool)"] -> w560
                  tunnel: [FALSE FALSE TRUE FALSE FALSE] -> w557
                  frame 0, Default {
                  }
                  frame 1 {
                  }
                  frame 2 {
                  }
                  frame 3 {
                  }
                  frame 4 {
                  }
                }
                n308 = case shown="False" w543 {
                  tunnel: ["No" "Yes"] -> w541
                  frame False {
                  }
                  frame True {
                  }
                }
                n309 = case shown="True" w544 {
                  tunnel: ["Skip" "Run"] -> w542
                  frame False {
                  }
                  frame True {
                  }
                }
                n310 = Number To Decimal String(number=w562) -> (decimal integer string=w561:string)  [unwired: 1 in]
                n311 = Number To Decimal String(number=w549) -> (decimal integer string=w540:string)  [unwired: 1 in]
                n312 = case shown="\"Idle\", Default" w553 {
                  tunnel: ["Idle" "PASS" "FALSE"] -> w552
                  frame "Idle", Default {
                  }
                  frame "PASS" {
                  }
                  frame "FALSE" {
                  }
                }
                n313 = Concatenate Strings(w561, w560) -> (w559:string)
                n314 = case shown="True" w557 {
                  tunnel: [w575 w584] -> w550
                  tunnel: [w575 w581] -> w555
                  tunnel: w556 -> [_ w579]
                  tunnel: w546 -> [_ w578]
                  tunnel: w545 -> [_ w577]
                  tunnel: w551 -> [_ w576]
                  frame False {
                    w575 = "..."
                  }
                  frame True {
                    n315 = Format Into String(format string="%5.2f", w578) -> (resulting string=w586:string)  [unwired: 2 in, 1 out]
                    n316 = Format Into String(format string="%5.2f", w577) -> (resulting string=w585:string)  [unwired: 2 in, 1 out]
                    n317 = Format Into String(format string="%5.2f", w579) -> (resulting string=w583:string)  [unwired: 2 in, 1 out]
                    n318 = Concatenate Strings(w586, "\r", w585) -> (w584:string)
                    n319 = Concatenate Strings(w583, " (", w576, ")") -> (w581:string)
                  }
                }
                n320 = property on="Test Sequencer" class="MCListbox (strict)"() -> ("ItemNames"=w565:string[][])  [unwired: 2 in, 2 out]
                n321 = Build Array(w559, w558, w555, w554, w550, w552, w542, w547, w540, w541) -> (w563:string[])
                n322 = Replace Array Subset(array=w565, new element=w563, index (row)=w562) -> (w564:string[][])  [unwired: 1 in]
                n323 = property on="Test Sequencer" class="MCListbox (strict)"("ItemNames"=w564) -> ()  [unwired: 2 in, 2 out]
              }
            }
            frame #2 {
              n324 = local read "Row Selected"() -> (w601:i16)
              n325 = disable-structure shown="Disabled" {
                disable-tunnel: w601 -> [w602 _]
                frame Disabled {
                  n326 = in-place {
                    in-place-border: w602 -> [w605]
                    w607 = 10 ("y")
                    # "Update Scrool Bar"
                    # "Rows on List Box"
                    n327 = Increment(x=w605) -> (x+1=w604:i16)
                    n328 = Greater?(x=w604, y=w607) -> (0:w610:bool)
                    n329 = Subtract(x=w604, y=w607) -> (x-y=w608:i32)
                    n330 = Select(t=w608, s=w610, f=0) -> (s? t:f=w606:i32)
                    n331 = Bundle By Name(cluster=T4 {"Row"=0, "Column"=0} ("Top Left Visible Cell"), "Row"=w606) -> (w603:T4)
                    n332 = property on="Test Sequencer" class="MCListbox (strict)"("TopLeft"=w603) -> ()  [unwired: 2 in, 2 out]
                  }
                }
                frame Enabled {
                }
              }
              n333 = property on="Test Sequencer" class="MCListbox (strict)"("Value"=w601) -> ()  [unwired: 2 in, 2 out]
            }
          }
        }
        event "Replace Step": Value Change {
          n334 = event-data() -> ()  [unwired: 1 in, 6 out]
          n335 = flat-sequence {
            tunnel: [w626] -> w617
            tunnel: [w624] -> w616
            tunnel: [w622] -> w615
            tunnel: [w620] -> w614
            tunnel: [w618] -> w613
            tunnel: w617 -> [w670]
            tunnel: w616 -> [w665]
            tunnel: w615 -> [w660]
            tunnel: [w658] -> w612
            tunnel: w614 -> [w659]
            tunnel: w613 -> [w658]
            tunnel: w612 -> [w691]
            frame #0 {
              n336 = local read "Step-ID"() -> (w639:u16)
              n337 = local read "Description"() -> (w638:string)
              n338 = local read "Step Type"() -> (w636:T2)
              n339 = local read "Parameters"() -> (w637:string)
              n340 = local read "Run/Skip"() -> (w635:bool)
              n341 = local read "Report"() -> (w634:bool)
              n342 = local read "Measure Units"() -> (w633:string)
              n343 = local read "Value Nominal"() -> (w621:dbl)
              n344 = local read "Upper Limt"() -> (w632:dbl)
              n345 = local read "Lower Limt"() -> (w631:dbl)
              n346 = Bundle By Name(cluster=T5 {"Step ID"=0, "Step Description"="", "Step Type"=0, "Test Values"={"Numeric Value"=0.0, "Str Value"="", "Boolean Value"=TRUE, "Upper Limit"=0.0, "Lower Limit"=0.0}, "Parameters"="", "Run/Skip"=TRUE, "Test Result"=enum."Idle", "Report"=TRUE, "Measure Units"="..."} ("Test Step"), "Step ID"=w639, "Step Description"=w638, "Step Type"=w636, "Parameters"=w637, "Run/Skip"=w635, "Report"=w634, "Measure Units"=w633, "Test Values.Numeric Value"=w621, "Test Values.Str Value"="...", "Test Values.Boolean Value"=TRUE, "Test Values.Upper Limit"=w632, "Test Values.Lower Limit"=w631, "Test Result"=Test_Result."Idle") -> (w640:T5)
              n347 = local read "Row Selected"() -> (w618:i16)
              n348 = global read "Sequencer Array.vi" "SEQUENCER Array"() -> (w642:T5[])
              n349 = local read "Run/Skip"() -> (w625:bool)
              n350 = Replace Array Subset(array=w642, new element=w640, index=w618) -> (w641:T5[])
              n351 = local read "Step Type"() -> (w627:T2)
              n352 = local read "Report"() -> (w623:bool)
              n353 = global write "Sequencer Array.vi" "SEQUENCER Array"(w641) -> ()
              n354 = case shown="True" w625 {
                tunnel: ["Skip" "Run"] -> w624
                frame False {
                }
                frame True {
                }
              }
              n355 = case shown="False" w623 {
                tunnel: ["No" "Yes"] -> w622
                frame False {
                }
                frame True {
                }
              }
              n356 = case shown="3" w627 {
                tunnel: ["- (Label)" "- (Sets)" "- (Numer)" "- (String)" "- (Bool)"] -> w626
                tunnel: [FALSE FALSE TRUE FALSE FALSE] -> w620
                frame 0, Default {
                }
                frame 1 {
                }
                frame 2 {
                }
                frame 3 {
                }
                frame 4 {
                }
              }
            }
            frame #1 {
              # "Update Test Seqiencer Box"
              n357 = case shown="True" w659 {
                tunnel: [w675 w682] -> w667
                tunnel: [w675 w679] -> w666
                frame False {
                  w675 = "..."
                }
                frame True {
                  n358 = local read "Value Nominal"() -> (w676:dbl)
                  n359 = local read "Measure Units"() -> (w678:string)
                  n360 = local read "Lower Limt"() -> (w686:dbl)
                  n361 = local read "Upper Limt"() -> (w688:dbl)
                  n362 = Format Into String(format string="%5.2f", w688) -> (resulting string=w684:string)  [unwired: 2 in, 1 out]
                  n363 = Format Into String(format string="%5.2f", w686) -> (resulting string=w683:string)  [unwired: 2 in, 1 out]
                  n364 = Format Into String(format string="%5.2f", w676) -> (resulting string=w681:string)  [unwired: 2 in, 1 out]
                  n365 = Concatenate Strings(w684, "\r", w683) -> (w682:string)
                  n366 = Concatenate Strings(w681, " (", w678, ")") -> (w679:string)
                }
              }
              n367 = Number To Decimal String(number=w658) -> (decimal integer string=w671:string)  [unwired: 1 in]
              n368 = local read "Step-ID"() -> (w663:u16)
              n369 = Concatenate Strings(w671, w670) -> (w669:string)
              n370 = Number To Decimal String(number=w663) -> (decimal integer string=w661:string)  [unwired: 1 in]
              n371 = local read "Description"() -> (w668:string)
              n372 = local read "Parameters"() -> (w664:string)
              n373 = property on="Test Sequencer" class="MCListbox (strict)"() -> ("ItemNames"=w674:string[][])  [unwired: 2 in, 2 out]
              n374 = Build Array(w669, w668, w666, "...", w667, "Idle", w665, w664, w661, w660) -> (w672:string[])
              n375 = Replace Array Subset(array=w674, new element=w672, index (row)=w658) -> (w673:string[][])  [unwired: 1 in]
              n376 = property on="Test Sequencer" class="MCListbox (strict)"("ItemNames"=w673) -> ()  [unwired: 2 in, 2 out]
            }
            frame #2 {
              n377 = disable-structure shown="Disabled" {
                disable-tunnel: w691 -> [w694 _]
                frame Disabled {
                  n378 = in-place {
                    in-place-border: w694 -> [w697]
                    w699 = 10 ("y")
                    # "Update Scrool Bar"
                    # "Rows on List Box"
                    n379 = Increment(x=w697) -> (x+1=w696:i16)
                    n380 = Greater?(x=w696, y=w699) -> (0:w702:bool)
                    n381 = Subtract(x=w696, y=w699) -> (x-y=w700:i32)
                    n382 = Select(t=w700, s=w702, f=0) -> (s? t:f=w698:i32)
                    n383 = Bundle By Name(cluster=T4 {"Row"=0, "Column"=0} ("Top Left Visible Cell"), "Row"=w698) -> (w695:T4)
                    n384 = property on="Test Sequencer" class="MCListbox (strict)"("TopLeft"=w695) -> ()  [unwired: 2 in, 2 out]
                  }
                }
                frame Enabled {
                }
              }
              n385 = local write "Row Selected"(w691) -> ()
              n386 = property on="Test Sequencer" class="MCListbox (strict)"("Value"=w691) -> ()  [unwired: 2 in, 2 out]
              n387 = global read "Sequencer Array.vi" "SEQUENCER Array"() -> (w693:T5[])
              n388 = Array Size(array=w693) -> (size(s)=w692:i32)
              n389 = local write "Steps"(w692) -> ()
            }
          }
        }
        event Double Click {
          n390 = event-data() -> ("Row"=w704:i32)  [unwired: 1 in, 8 out]
          n391 = flat-sequence {
            tunnel: w704 -> [w707]
            frame #0 {
              n392 = local read "Steps"() -> (w706:u16)
              n393 = Greater Or Equal?(x=w707, y=w706) -> (x >= y?=w705:bool)
              n394 = case shown="True" w705 {
                tunnel: w707 -> [w708 _]
                frame False {
                  n395 = property on="Test Sequencer" class="MCListbox (strict)"("Value"=w708) -> ()  [unwired: 2 in, 2 out]
                  n396 = local write "Row Selected"(w708) -> ()
                }
                frame True {
                  n397 = local read "Steps"() -> (w710:u16)
                  n398 = Decrement(x=w710) -> (x-1=w709:u16)
                  n399 = in-place {
                    in-place-border: w709 -> [w714]
                    in-place-border: [w711] -> _
                    w716 = 7 ("y")
                    # "Update Scrool Bar"
                    # "Rows on List Box"
                    n400 = Increment(x=w714) -> (x+1=w713:u16)
                    n401 = Greater?(x=w713, y=w716) -> (0:w719:bool)
                    n402 = Subtract(x=w713, y=w716) -> (x-y=w717:i32)
                    n403 = Select(t=w717, s=w719, f=0) -> (s? t:f=w715:i32)
                    n404 = Bundle By Name(cluster=T4 {"Row"=0, "Column"=0} ("Top Left Visible Cell"), "Row"=w715) -> (w712:T4)
                    n405 = property on="Test Sequencer" class="MCListbox (strict)"("TopLeft"=w712) -> (error out=w711:errorcluster)  [unwired: 2 in, 1 out]
                  }
                  n406 = property on="Test Sequencer" class="MCListbox (strict)"("Value"=w709) -> ()  [unwired: 2 in, 2 out]
                  n407 = local write "Row Selected"(w709) -> ()
                }
              }
            }
            frame #1 {
              n408 = local read "Row Selected"() -> (w721:i16)
              n409 = global read "Sequencer Array.vi" "SEQUENCER Array"() -> (w722:T5[])
              n410 = Array Size(array=w722) -> (size(s)=w724:i32)
              n411 = Greater Than 0?(x=w724) -> (x > 0?=w723:bool)
              n412 = case shown="True" w723 {
                tunnel: w722 -> [_ w737]
                tunnel: w721 -> [_ w736]
                frame False {
                }
                frame True {
                  n413 = Index Array(array=w737, index=w736) -> (element=w735:T5)
                  n414 = Unbundle By Name(w735) -> ("Step ID"=w734:u16, "Step Description"=w732:string, "Step Type"=w733:u16, "Measure Units"=w725:string, "Parameters"=w729:string, "Run/Skip"=w731:bool, "Report"=w730:bool, "Test Values.Numeric Value"=w728:dbl, "Test Values.Upper Limit"=w727:dbl, "Test Values.Lower Limit"=w726:dbl)  [unwired: 1 out]
                  n415 = local write "Step-ID"(w734) -> ()
                  n416 = local write "Step Type"(w733) -> ()
                  n417 = local write "Run/Skip"(w731) -> ()
                  n418 = local write "Report"(w730) -> ()
                  n419 = local write "Value Nominal"(w728) -> ()
                  n420 = local write "Upper Limt"(w727) -> ()
                  n421 = local write "Lower Limt"(w726) -> ()
                  n422 = local write "Parameters"(w729) -> ()
                  n423 = local write "Description"(w732) -> ()
                  n424 = local write "Measure Units"(w725) -> ()
                }
              }
            }
          }
        }
        event "Remove Step": Value Change {
          n425 = event-data() -> ()  [unwired: 1 in, 6 out]
          n426 = flat-sequence {
            tunnel: [w739] -> w738
            tunnel: w738 -> [w757]
            frame #0 {
              n427 = global read "Sequencer Array.vi" "SEQUENCER Array"() -> (w742:T5[])
              n428 = in-place {
                # "Reinit Test Sequencer"
                n429 = Initialize Array("", 250, 10 ("dimension size")) -> (w754:string[][])
                n430 = property on="Test Sequencer" class="MCListbox (strict)"("ItemNames"=w754, "TopLeft"=T4 {"Row"=0, "Column"=0} ("Top Left Visible Cell"), "Value"=T1 0 ("Test Sequencer")) -> ()  [unwired: 2 in, 2 out]
              }
              n431 = Array Size(array=w742) -> (size(s)=w740:i32)
              n432 = Greater Than 0?(x=w740) -> (x > 0?=w741:bool)
              n433 = case shown="True" w741 {
                tunnel: [0 w745] -> w739
                frame False {
                  n434 = local write "Steps"(u16 0 ("Steps")) -> ()
                }
                frame True {
                  n435 = global read "Sequencer Array.vi" "SEQUENCER Array"() -> (w750:T5[])
                  n436 = local read "Row Selected"() -> (w748:i16)
                  n437 = Delete From Array(array=w750, length=1, index=w748) -> (array with subset deleted=w746:T5[])  [unwired: 1 out]
                  n438 = Decrement(x=w748) -> (x-1=w747:i16)
                  n439 = Array Size(array=w746) -> (size(s)=w745:i32)
                  n440 = global write "Sequencer Array.vi" "SEQUENCER Array"(w746) -> ()
                  n441 = local write "Row Selected"(w747) -> ()
                  n442 = local write "Steps"(w745) -> ()
                }
              }
            }
            frame #1 {
              n443 = for {
                N: w757 -> [_]
                i -> [w780]
                # "Revrite Table"
                n444 = global read "Sequencer Array.vi" "SEQUENCER Array"() -> (w785:T5[])
                n445 = Index Array(array=w785, index=w780) -> (element=w766:T5)
                n446 = Unbundle By Name(w766) -> ("Step Type"=w784:u16, "Step Description"=w776:string, "Test Values.Str Value"=w772:string, "Test Result"=w771:T6, "Measure Units"=w769:string, "Parameters"=w765:string, "Step ID"=w767:u16, "Test Values.Numeric Value"=w774:dbl, "Test Values.Upper Limit"=w764:dbl, "Test Values.Lower Limit"=w763:dbl, "Run/Skip"=w762:bool, "Report"=w761:bool)  [unwired: 1 out]
                n447 = case shown="2" w784 {
                  tunnel: ["- (Label)" "- (Sets)" "- (Numer)" "- (String)" "- (Bool)"] -> w778
                  tunnel: [FALSE FALSE TRUE FALSE FALSE] -> w775
                  frame 0, Default {
                  }
                  frame 1 {
                  }
                  frame 2 {
                  }
                  frame 3 {
                  }
                  frame 4 {
                  }
                }
                n448 = case shown="False" w761 {
                  tunnel: ["No" "Yes"] -> w759
                  frame False {
                  }
                  frame True {
                  }
                }
                n449 = case shown="True" w762 {
                  tunnel: ["Skip" "Run"] -> w760
                  frame False {
                  }
                  frame True {
                  }
                }
                n450 = Number To Decimal String(number=w780) -> (decimal integer string=w779:string)  [unwired: 1 in]
                n451 = Number To Decimal String(number=w767) -> (decimal integer string=w758:string)  [unwired: 1 in]
                n452 = case shown="\"Idle\", Default" w771 {
                  tunnel: ["Idle" "PASS" "FALSE"] -> w770
                  frame "Idle", Default {
                  }
                  frame "PASS" {
                  }
                  frame "FALSE" {
                  }
                }
                n453 = Concatenate Strings(w779, w778) -> (w777:string)
                n454 = case shown="True" w775 {
                  tunnel: [w793 w802] -> w768
                  tunnel: [w793 w799] -> w773
                  tunnel: w774 -> [_ w797]
                  tunnel: w764 -> [_ w796]
                  tunnel: w763 -> [_ w795]
                  tunnel: w769 -> [_ w794]
                  frame False {
                    w793 = "..."
                  }
                  frame True {
                    n455 = Format Into String(format string="%5.2f", w796) -> (resulting string=w804:string)  [unwired: 2 in, 1 out]
                    n456 = Format Into String(format string="%5.2f", w795) -> (resulting string=w803:string)  [unwired: 2 in, 1 out]
                    n457 = Format Into String(format string="%5.2f", w797) -> (resulting string=w801:string)  [unwired: 2 in, 1 out]
                    n458 = Concatenate Strings(w804, "\r", w803) -> (w802:string)
                    n459 = Concatenate Strings(w801, "(", w794, ")") -> (w799:string)
                  }
                }
                n460 = property on="Test Sequencer" class="MCListbox (strict)"() -> ("ItemNames"=w783:string[][])  [unwired: 2 in, 2 out]
                n461 = Build Array(w777, w776, w773, w772, w768, w770, w760, w765, w758, w759) -> (w781:string[])
                n462 = Replace Array Subset(array=w783, new element=w781, index (row)=w780) -> (w782:string[][])  [unwired: 1 in]
                n463 = property on="Test Sequencer" class="MCListbox (strict)"("ItemNames"=w782) -> ()  [unwired: 2 in, 2 out]
              }
            }
            frame #2 {
              n464 = local read "Row Selected"() -> (w819:i16)
              n465 = in-place {
                in-place-border: w819 -> [w822]
                w824 = 10 ("y")
                # "Update Scrool Bar"
                # "Rows on List Box"
                n466 = Increment(x=w822) -> (x+1=w821:i16)
                n467 = Greater?(x=w821, y=w824) -> (0:w827:bool)
                n468 = Subtract(x=w821, y=w824) -> (x-y=w825:i32)
                n469 = Select(t=w825, s=w827, f=0) -> (s? t:f=w823:i32)
                n470 = Bundle By Name(cluster=T4 {"Row"=0, "Column"=0} ("Top Left Visible Cell"), "Row"=w823) -> (w820:T4)
                n471 = property on="Test Sequencer" class="MCListbox (strict)"("TopLeft"=w820) -> ()  [unwired: 2 in, 2 out]
              }
              n472 = property on="Test Sequencer" class="MCListbox (strict)"("Value"=w819) -> ()  [unwired: 2 in, 2 out]
            }
          }
        }
        event "Clear Array": Value Change {
          n473 = event-data() -> ()  [unwired: 1 in, 6 out]
          n474 = flat-sequence {
            frame #0 {
              w830 = 0.0
              w829 = ""
              w835 = u16 0 ("Steps")
              n475 = global read "Sequencer Array.vi" "SEQUENCER Array"() -> (w838:T5[])
              n476 = local write "Prc % (+)"(5) -> ()
              n477 = local write "Prc % (-)"(i16 -5 ("Prc % (-)")) -> ()
              n478 = local write "Steps"(w835) -> ()
              n479 = local write "Row Selected"(w835) -> ()
              n480 = property on="Parameters" class="Str"("Value"=w829) -> ()  [unwired: 2 in, 2 out]
              n481 = property on="Description" class="Str"("Value"=w829) -> ()  [unwired: 2 in, 2 out]
              n482 = Array Size(array=w838) -> (size(s)=w837:i32)
              n483 = local write "Run/Skip"(FALSE ("Run/Skip")) -> ()
              n484 = local write "Report"(FALSE ("Report")) -> ()
              n485 = local write "Value Nominal"(w830) -> ()
              n486 = local write "Upper Limt"(w830) -> ()
              n487 = local write "Lower Limt"(w830) -> ()
              n488 = Delete From Array(array=w838, length=w837) -> (array with subset deleted=w836:T5[])  [unwired: 1 in, 1 out]
              n489 = global write "Sequencer Array.vi" "SEQUENCER Array"(w836) -> ()
            }
            frame #1 {
              n490 = in-place "In Place Element Structure" {
                # "Cleare Sequencer Table"
                n491 = control-ref of="Test Sequencer"() -> (w840:refnum<vi>)
                n492 = Initialize Array("", 250 ("dimension size"), 10 ("dimension size")) -> (w843:string[][])
                n493 = property on="Property Node" class="MCListbox (strict)"(reference=w840, "ItemNames"=w843, "TopLeft"=T4 {"Row"=0, "Column"=0} ("Top Left Visible Cell"), "Value"=T1 0 ("Test Sequencer")) -> ()  [unwired: 1 in, 2 out]
              }
            }
          }
        }
        event "New Step": Value Change {
          n494 = event-data() -> ()  [unwired: 1 in, 6 out]
          n495 = flat-sequence {
            tunnel: [w860] -> w851
            tunnel: [w858] -> w850
            tunnel: [w856] -> w849
            tunnel: [w854] -> w847
            tunnel: [w853] -> w846
            tunnel: w851 -> [w904]
            tunnel: w850 -> [w899]
            tunnel: w849 -> [w894]
            tunnel: [w892] -> w848
            tunnel: w847 -> [w893]
            tunnel: w846 -> [w892]
            tunnel: w848 -> [w925]
            frame #0 {
              n496 = local read "Step-ID"() -> (w873:u16)
              n497 = local read "Description"() -> (w872:string)
              n498 = local read "Step Type"() -> (w870:T2)
              n499 = local read "Parameters"() -> (w871:string)
              n500 = local read "Run/Skip"() -> (w869:bool)
              n501 = local read "Report"() -> (w868:bool)
              n502 = local read "Measure Units"() -> (w867:string)
              n503 = local read "Value Nominal"() -> (w855:dbl)
              n504 = local read "Upper Limt"() -> (w866:dbl)
              n505 = local read "Lower Limt"() -> (w865:dbl)
              n506 = Bundle By Name(cluster=T5 {"Step ID"=0, "Step Description"="", "Step Type"=0, "Test Values"={"Numeric Value"=0.0, "Str Value"="", "Boolean Value"=TRUE, "Upper Limit"=0.0, "Lower Limit"=0.0}, "Parameters"="", "Run/Skip"=TRUE, "Test Result"=enum."Idle", "Report"=TRUE, "Measure Units"="..."} ("Test Step"), "Step ID"=w873, "Step Description"=w872, "Step Type"=w870, "Parameters"=w871, "Run/Skip"=w869, "Report"=w868, "Measure Units"=w867, "Test Values.Numeric Value"=w855, "Test Values.Str Value"="<...>", "Test Values.Boolean Value"=TRUE, "Test Values.Upper Limit"=w866, "Test Values.Lower Limit"=w865, "Test Result"=Test_Result."Idle") -> (w874:T5)
              n507 = global read "Sequencer Array.vi" "SEQUENCER Array"() -> (w876:T5[])
              n508 = local read "Steps"() -> (w853:u16)
              n509 = local read "Run/Skip"() -> (w859:bool)
              n510 = Insert Into Array(array=w876, index=w853, new element=w874) -> (w875:T5[])
              n511 = local read "Step Type"() -> (w861:T2)
              n512 = local read "Report"() -> (w857:bool)
              n513 = global write "Sequencer Array.vi" "SEQUENCER Array"(w875) -> ()
              n514 = case shown="True" w859 {
                tunnel: ["Skip" "Run"] -> w858
                frame False {
                }
                frame True {
                }
              }
              n515 = case shown="False" w857 {
                tunnel: ["No" "Yes"] -> w856
                frame False {
                }
                frame True {
                }
              }
              n516 = case shown="2" w861 {
                tunnel: ["- (Label)" "- (Sets)" "- (Numer)" "- (String)" "- (Bool)"] -> w860
                tunnel: [FALSE FALSE TRUE FALSE FALSE] -> w854
                frame 0, Default {
                }
                frame 1 {
                }
                frame 2 {
                }
                frame 3 {
                }
                frame 4 {
                }
              }
            }
            frame #1 {
              # "Update Test Seqiencer Box"
              n517 = case shown="True" w893 {
                tunnel: [w909 w916] -> w901
                tunnel: [w909 w913] -> w900
                frame False {
                  w909 = ""
                  (unwired) "..."
                }
                frame True {
                  n518 = local read "Value Nominal"() -> (w910:dbl)
                  n519 = local read "Measure Units"() -> (w912:string)
                  n520 = local read "Lower Limt"() -> (w920:dbl)
                  n521 = local read "Upper Limt"() -> (w922:dbl)
                  n522 = Format Into String(format string="%5.2f", w922) -> (resulting string=w918:string)  [unwired: 2 in, 1 out]
                  n523 = Format Into String(format string="%5.2f", w920) -> (resulting string=w917:string)  [unwired: 2 in, 1 out]
                  n524 = Format Into String(format string="%5.2f", w910) -> (resulting string=w915:string)  [unwired: 2 in, 1 out]
                  n525 = Concatenate Strings(w918, "\r", w917) -> (w916:string)
                  n526 = Concatenate Strings(w915, " (", w912, ")") -> (w913:string)
                }
              }
              n527 = Number To Decimal String(number=w892) -> (decimal integer string=w905:string)  [unwired: 1 in]
              n528 = local read "Step-ID"() -> (w897:u16)
              n529 = Concatenate Strings(w905, w904) -> (w903:string)
              n530 = Number To Decimal String(number=w897) -> (decimal integer string=w895:string)  [unwired: 1 in]
              n531 = local read "Description"() -> (w902:string)
              n532 = local read "Parameters"() -> (w898:string)
              n533 = property on="Test Sequencer" class="MCListbox (strict)"() -> ("ItemNames"=w908:string[][])  [unwired: 2 in, 2 out]
              n534 = Build Array(w903, w902, w900, "<...>", w901, "Idle", w899, w898, w895, w894) -> (w906:string[])
              n535 = Replace Array Subset(array=w908, new element=w906, index (row)=w892) -> (w907:string[][])  [unwired: 1 in]
              n536 = property on="Test Sequencer" class="MCListbox (strict)"("ItemNames"=w907) -> ()  [unwired: 2 in, 2 out]
            }
            frame #2 {
              n537 = local write "Row Selected"(w925) -> ()
              n538 = in-place {
                in-place-border: w925 -> [w930]
                in-place-border: [w929] -> _
                w932 = 10 ("y")
                # "Update Scrool Bar"
                # "Rows on List Box"
                n539 = Increment(x=w930) -> (x+1=w929:u16)
                n540 = Greater?(x=w929, y=w932) -> (0:w935:bool)
                n541 = Subtract(x=w929, y=w932) -> (x-y=w933:i32)
                n542 = Select(t=w933, s=w935, f=0) -> (s? t:f=w931:i32)
                n543 = Bundle By Name(cluster=T4 {"Row"=0, "Column"=0} ("Top Left Visible Cell"), "Row"=w931) -> (w928:T4)
                n544 = property on="Test Sequencer" class="MCListbox (strict)"("TopLeft"=w928) -> ()  [unwired: 2 in, 2 out]
              }
              n545 = property on="Test Sequencer" class="MCListbox (strict)"("Value"=w925) -> ()  [unwired: 2 in, 2 out]
              n546 = global read "Sequencer Array.vi" "SEQUENCER Array"() -> (w927:T5[])
              n547 = Array Size(array=w927) -> (size(s)=w926:i32)
              n548 = local write "Steps"(w926) -> ()
            }
          }
        }
      }
    }
  }
